vi "Initialize.vi"(8 "error in":errorcluster, 10 "parameters":variant, 11 "Fgen Channel in":refnum<class "Fgen Channel.lvclass">) -> (0 "error out":errorcluster, 2 "summary":T2[](array[typedef]), 3 "data value reference":T1)   [LabVIEW 2025, in "Fgen.lvlib" / "Fgen Channel.lvclass"]
doc: "This Vi initializes the data of a node its default state.\nThe object is not created inside of this ViI, beacuase it is created from a File depending on user selection.Copyright 2017 National Instruments Corporation\n\nLicensed under the Apache License, Version 2.0 (the \"License\"); you may not use this file except in compliance with the License. You may obtain a copy of the License at http://www.apache.org/licenses/LICENSE-2.0\nUnless required by applicable law or agreed to in writing, software distributed under the License is distributed on an \"AS IS\" BASIS, WITHOUT WARRANTIES OR CONDITIONS OF ANY KIND, either express or implied. See the License for the specific language governing permissions and limitations under the License."
uses:
  Fgen Channel.lvclass
  C:/Users/Public/Documents/Sandia National Labs/TSS Plugin/CEF.lvlibp/Node/CEF_Node.lvclass
  Users/Public/Documents/Sandia National Labs/TSS Plugin/CEF.lvlibp/Node/Summary.ctl
  Users/Public/Documents/Sandia National Labs/TSS Plugin/CEF.lvlibp/Node/NodeRef.ctl
  Users/Public/Documents/Sandia National Labs/TSS Plugin/CEF.lvlibp/Node/CEF_Node.lvclass
  Fgen Instrument/Fgen Instrument.lvclass
  Fgen Channel.lvclass/Fgen Channel.ctl
  Fgen configuration/Fgen configuration.lvclass
  C:/Users/Public/Documents/Sandia National Labs/TSS Plugin/Abstract Engine.lvlibp/Instrument configuration/Instrument configuration.lvclass
  Fgen Channel configuration/Fgen Channel configuration.lvclass
  C:/Users/Public/Documents/Sandia National Labs/TSS Plugin/Abstract Engine.lvlibp/Channel configuration/Channel configuration.lvclass
  Users/Public/Documents/Sandia National Labs/TSS Plugin/CEF.lvlibp/Node/ReadParent.vi
  Users/Public/Documents/Sandia National Labs/TSS Plugin/CEF.lvlibp/Node/ReadChildren.vi
  Users/Public/Documents/Sandia National Labs/TSS Plugin/Abstract Engine.lvlibp/Instrument configuration/Read Instrument Setting.vi
  Users/Public/Documents/Sandia National Labs/TSS Plugin/Abstract Engine.lvlibp/Channel configuration/Read Channel Setting.vi
  Users/Public/Documents/Sandia National Labs/TSS Plugin/Abstract Engine.lvlibp/Channel configuration/Write Channel Setting.vi
  Users/Public/Documents/Sandia National Labs/TSS Plugin/CEF.lvlibp/serializable configuration/CEF_serializable configuration.lvclass
  Users/Public/Documents/Sandia National Labs/TSS Plugin/Abstract Engine.lvlibp/Abstract Channel/Abstract Channel.lvclass
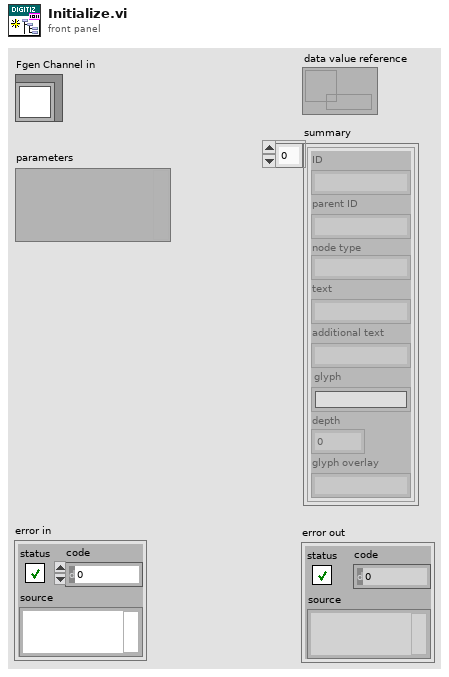
[diagram p1: front panel]
types:
  T1 = typedef "CEF.lvlibp/CEF_Node.lvclass/NodeRef.ctl" = refnum<data-value>
  T2 = typedef "CEF.lvlibp/CEF_Node.lvclass/Summary.ctl" = cluster{"ID":string, "parent ID":string, "node type":string, "text":string, "additional text":string, "glyph":string, "depth":i32, "glyph overlay":string}
  T3 = typedef "Abstract Engine.lvlibp/Instrument configuration.lvclass/Default Instrument.ctl" = cluster{"Type":string, "Address":string, "SW Alias":string, "Description":string, "Enabled":bool}
  T4 = typedef "Abstract Engine.lvlibp/Channel configuration.lvclass/Default Channel.ctl" = cluster{"Address":string, "SW Alias":string, "Enabled":bool, "Type":string, "Description":string}
  T5 = cluster{"ID":string, "parent ID":string, "node type":string, "text":string, "additional text":string, "glyph":string, "depth":i32, "glyph overlay":string}[]
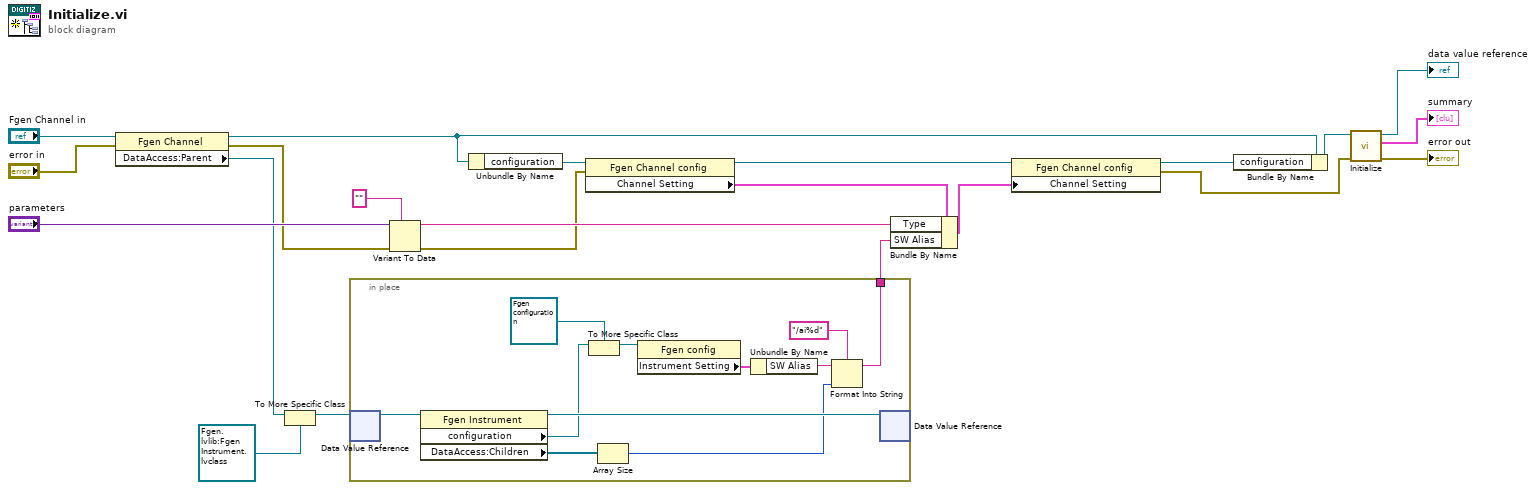
[diagram p0: block diagram]
diagram:
  n1 = property class="Fgen Channel"(reference="Fgen Channel in", error in="error in") -> (reference out=w14:refnum<class "Fgen Channel.lvclass">, error out=w8:errorcluster, "DataAccess:Parent"=w16:refnum<data-value>)
  n2 = To More Specific Class(target class=refnum<data-value> refnum ("data value reference"), reference=w16) -> (specific class reference=w17:refnum<data-value>)  [unwired: 1 in, 1 out]
  n3 = in-place {
    in-place-border: [w30] -> w9
    n4 = in-place-dvr #1(w17) -> (w29:refnum<class "Fgen Instrument.lvclass">)  [unwired: 1 out]
    n5 = property class="Fgen Instrument"(reference=w29) -> (reference out=w28:refnum<class "Fgen Instrument.lvclass">, "configuration"=w27:refnum<class "CEF_serializable configuration.lvclass">, "DataAccess:Children"=w26:refnum<data-value>[])  [unwired: 1 in, 1 out]
    n6 = To More Specific Class(target class=refnum<class "Fgen configuration.lvclass"> refnum ("Fgen.lvlib:Fgen configuration.lvclass"), reference=w27) -> (specific class reference=w33:refnum<class "Fgen configuration.lvclass">)  [unwired: 1 in, 1 out]
    n7 = Array Size(array=w26) -> (size(s)=w24:i32)
    n8 = property class="Fgen config"(reference=w33) -> ("Instrument Setting"=w23:T3)  [unwired: 1 in, 2 out]
    n9 = Unbundle By Name(w23) -> ("SW Alias"=w32:string)
    n10 = Format Into String(format string="/ai%d", initial string=w32, w24) -> (resulting string=w30:string)  [unwired: 1 in, 1 out]
    n11 = in-place-dvr #1(w28) -> ()  [unwired: 2 out]
  }
  n12 = Variant To Data(error in=w8, type="", Variant="parameters") -> (data=w7:string, error out=w5:errorcluster)
  n13 = Unbundle By Name(w14) -> ("configuration"=w15:refnum<class "Fgen Channel configuration.lvclass">)
  n14 = property class="Fgen Channel config"(reference=w15, error in=w5) -> (reference out=w10:refnum<class "Fgen Channel configuration.lvclass">, "Channel Setting"=w4:T4)  [unwired: 1 out]
  n15 = Bundle By Name(cluster=w4, "Type"=w7, "SW Alias"=w9) -> (w3:T4)
  n16 = property class="Fgen Channel config"(reference=w10, "Channel Setting"=w3) -> (reference out=w12:refnum<class "Fgen Channel configuration.lvclass">, error out=w2:errorcluster)  [unwired: 1 in]
  n17 = Bundle By Name(cluster=w14, "configuration"=w12) -> (w13:refnum<class "Fgen Channel.lvclass">)
  n18 = call-parent "Initialize.vi"("error in"=w2, "CEF_Serialize node in"=w13) -> ("error out"=→"error out":errorcluster, "summary"=→"summary":T5, "data value reference"=→"data value reference":refnum<data-value>)  [unwired: 7 in]
